vi "Modbus RTU Serial Request Translator.vi"(11 "请求字符串":string) -> (3 "转换后的字符串":string)   [LabVIEW 2014]
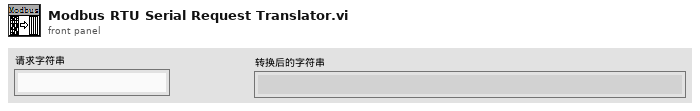
[diagram p1: front panel]
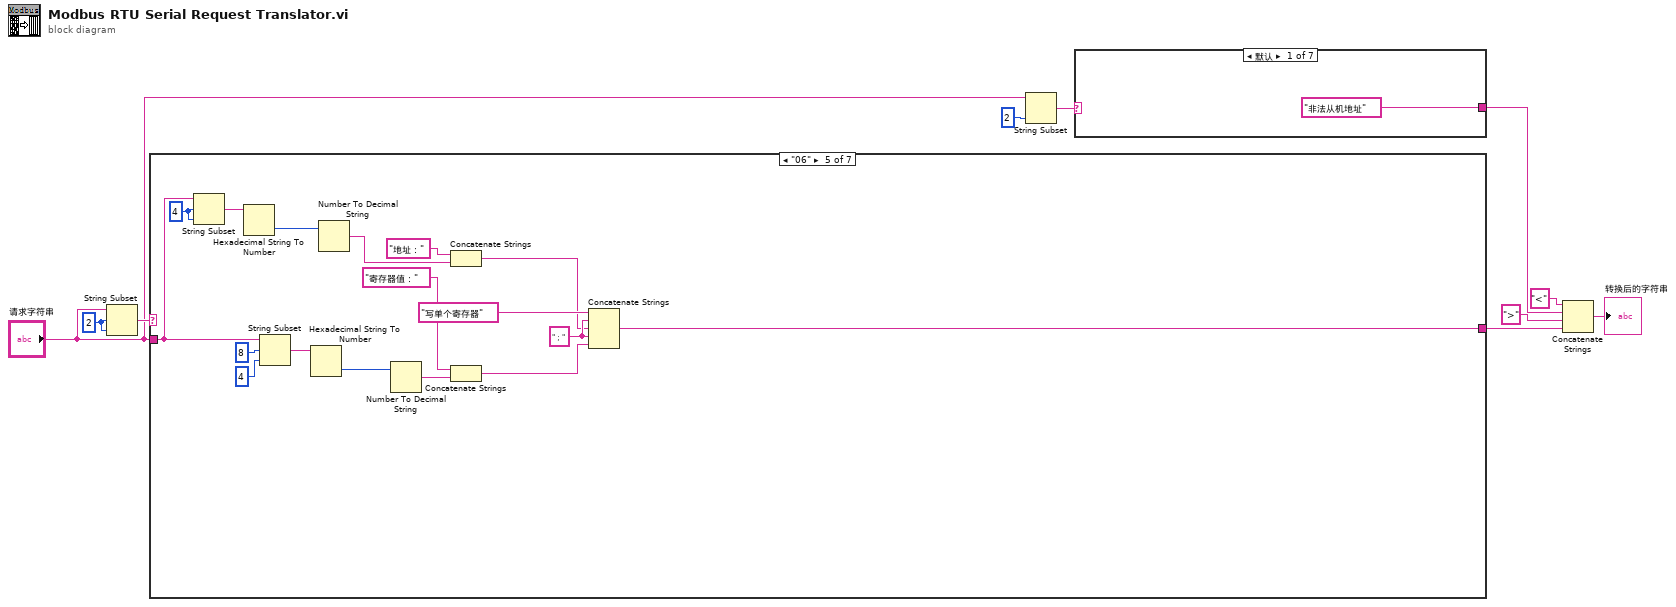
[diagram p0: block diagram]
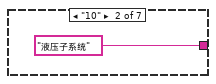
[diagram p2: hidden frame]
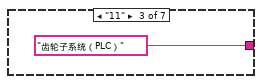
[diagram p3: hidden frame]
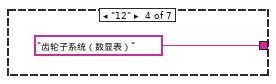
[diagram p4: hidden frame]
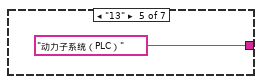
[diagram p5: hidden frame]
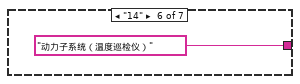
[diagram p6: hidden frame]
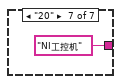
[diagram p7: hidden frame]
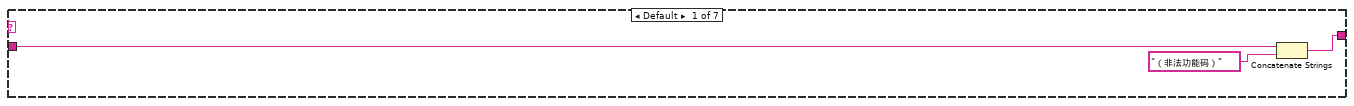
[diagram p8: hidden frame]
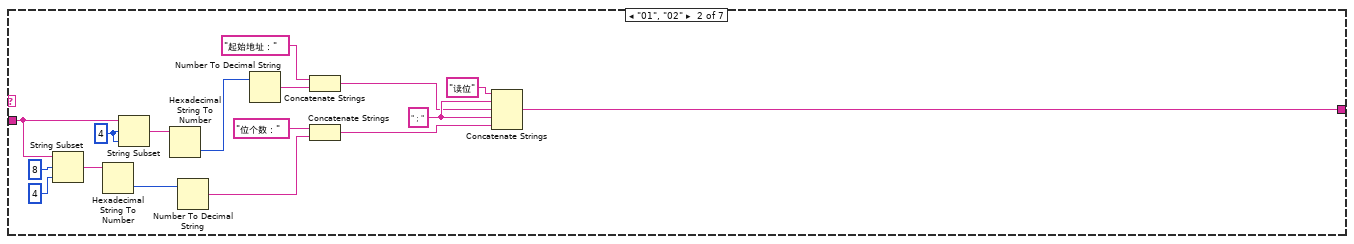
[diagram p9: hidden frame]
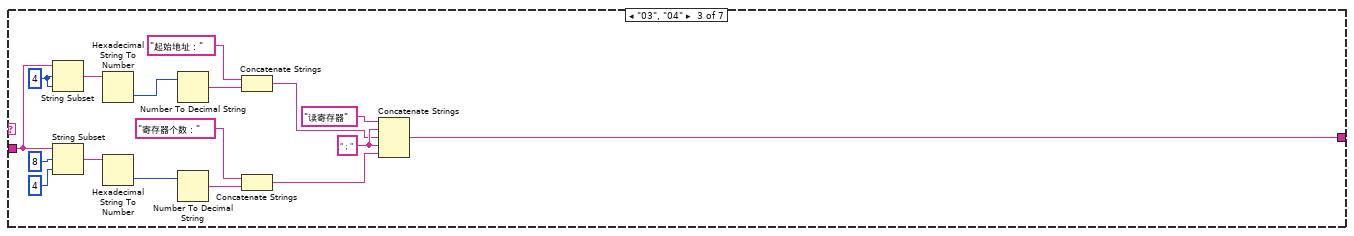
[diagram p10: hidden frame]
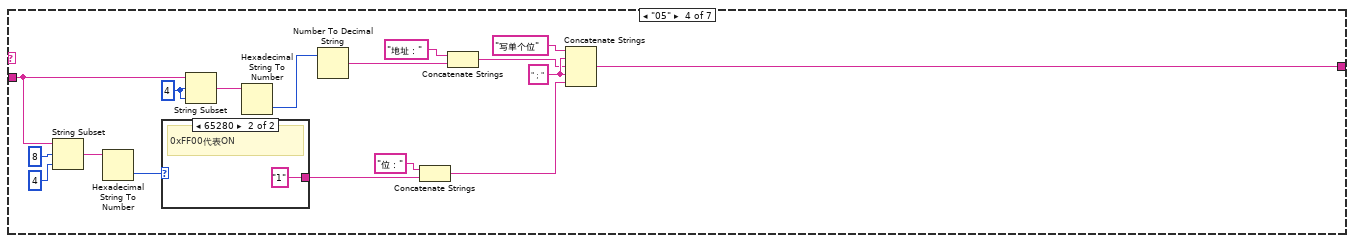
[diagram p11: hidden frame]
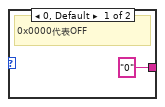
[diagram p12: hidden frame]
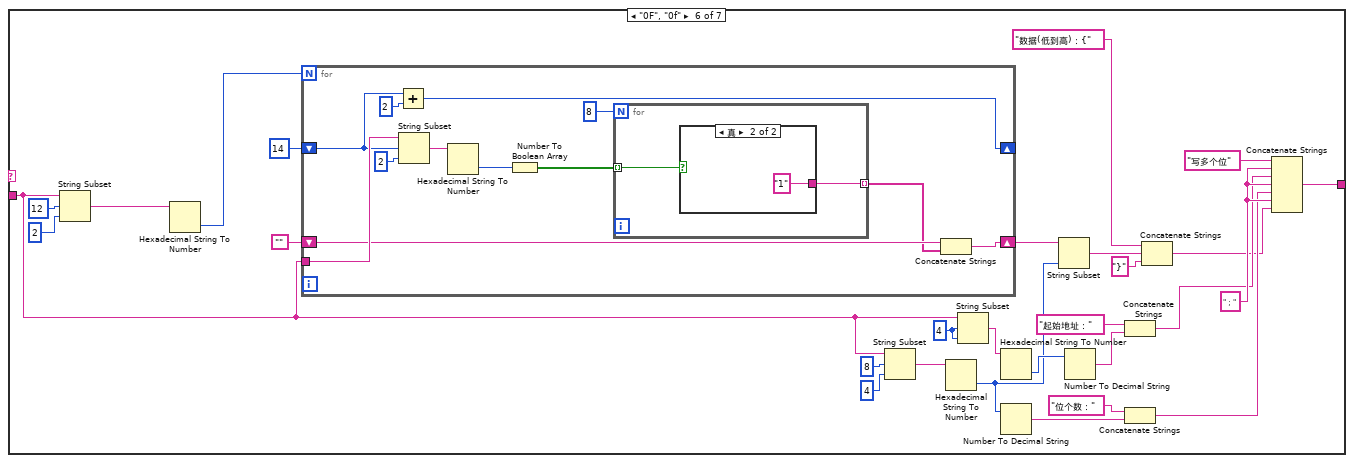
[diagram p13: hidden frame]
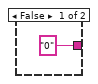
[diagram p14: hidden frame]
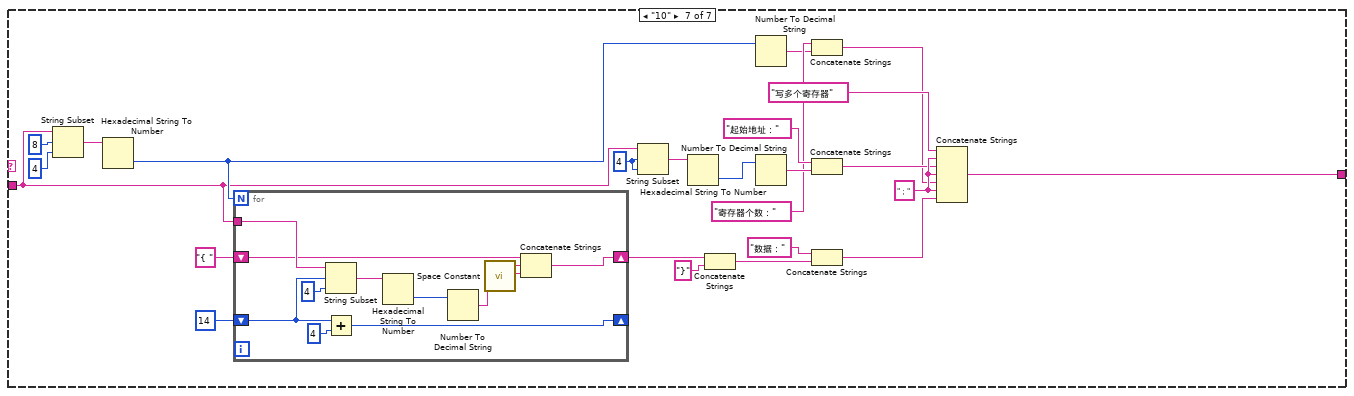
[diagram p15: hidden frame]
diagram:
  w10 = 2 ("偏移量(0)")
  n1 = String Subset(string="请求字符串", offset (0)=w10, length (rest)=w10) -> (substring=w9:string)
  n2 = case shown="\"06\"" w9 {
    tunnel: "请求字符串" -> [w13 w15 w46 w51 w72 w89 w143]
    tunnel: [w11 w14 w31 w50 w67 w94 w128] -> w5
    frame Default {
      n3 = Concatenate Strings(w13, "（非法功能码）") -> (w11:string)
    }
    frame "01", "02" {
      w18 = "；"
      w30 = 4 ("偏移量(0)")
      n4 = String Subset(string=w15, offset (0)=8 ("偏移量(0)"), length (rest)=4 ("长度（剩余）")) -> (substring=w21:string)
      n5 = Hexadecimal String To Number(string=w21) -> (number=w22:u32)  [unwired: 2 in, 1 out]
      n6 = String Subset(string=w15, offset (0)=w30, length (rest)=w30) -> (substring=w27:string)
      n7 = Hexadecimal String To Number(string=w27) -> (number=w26:u32)  [unwired: 2 in, 1 out]
      n8 = Number To Decimal String(number=w22) -> (decimal integer string=w20:string)  [unwired: 1 in]
      n9 = Number To Decimal String(number=w26) -> (decimal integer string=w24:string)  [unwired: 1 in]
      n10 = Concatenate Strings("起始地址：", w24) -> (w17:string)
      n11 = Concatenate Strings("位个数：", w20) -> (w16:string)
      n12 = Concatenate Strings("读位", w18, w17, w18, w16) -> (w14:string)
    }
    frame "03", "04" {
      w34 = "；"
      w47 = 4 ("偏移量(0)")
      n13 = String Subset(string=w46, offset (0)=w47, length (rest)=w47) -> (substring=w43:string)
      n14 = String Subset(string=w46, offset (0)=8 ("偏移量(0)"), length (rest)=4 ("长度（剩余）")) -> (substring=w37:string)
      n15 = Hexadecimal String To Number(string=w43) -> (number=w42:u32)  [unwired: 2 in, 1 out]
      n16 = Hexadecimal String To Number(string=w37) -> (number=w38:u32)  [unwired: 2 in, 1 out]
      n17 = Number To Decimal String(number=w42) -> (decimal integer string=w40:string)  [unwired: 1 in]
      n18 = Number To Decimal String(number=w38) -> (decimal integer string=w36:string)  [unwired: 1 in]
      n19 = Concatenate Strings("起始地址：", w40) -> (w33:string)
      n20 = Concatenate Strings("寄存器个数：", w36) -> (w32:string)
      n21 = Concatenate Strings("读寄存器", w34, w33, w34, w32) -> (w31:string)
    }
    frame "05" {
      w54 = "；"
      w64 = 4 ("偏移量(0)")
      n22 = String Subset(string=w51, offset (0)=8 ("偏移量(0)"), length (rest)=4 ("长度（剩余）")) -> (substring=w56:string)
      n23 = Hexadecimal String To Number(string=w56) -> (number=w49:u32)  [unwired: 2 in, 1 out]
      n24 = case shown="65280" w49 {
        tunnel: ["0" "1"] -> w48
        frame 0, Default {
          # "0x0000代表OFF"
        }
        frame 65280 {
          # "0xFF00代表ON"
        }
      }
      n25 = String Subset(string=w51, offset (0)=w64, length (rest)=w64) -> (substring=w61:string)
      n26 = Hexadecimal String To Number(string=w61) -> (number=w60:u32)  [unwired: 2 in, 1 out]
      n27 = Number To Decimal String(number=w60) -> (decimal integer string=w58:string)  [unwired: 1 in]
      n28 = Concatenate Strings("位：", w48) -> (w52:string)
      n29 = Concatenate Strings("地址：", w58) -> (w53:string)
      n30 = Concatenate Strings("写单个位", w54, w53, w54, w52) -> (w50:string)
    }
    frame "06" {
      w70 = "；"
      w83 = 4 ("偏移量(0)")
      n31 = String Subset(string=w72, offset (0)=w83, length (rest)=w83) -> (substring=w80:string)
      n32 = Hexadecimal String To Number(string=w80) -> (number=w79:u32)  [unwired: 2 in, 1 out]
      n33 = String Subset(string=w72, offset (0)=8 ("偏移量(0)"), length (rest)=4 ("长度（剩余）")) -> (substring=w74:string)
      n34 = Hexadecimal String To Number(string=w74) -> (number=w75:u32)  [unwired: 2 in, 1 out]
      n35 = Number To Decimal String(number=w79) -> (decimal integer string=w77:string)  [unwired: 1 in]
      n36 = Number To Decimal String(number=w75) -> (decimal integer string=w73:string)  [unwired: 1 in]
      n37 = Concatenate Strings("地址：", w77) -> (w69:string)
      n38 = Concatenate Strings("寄存器值：", w73) -> (w68:string)
      n39 = Concatenate Strings("写单个寄存器", w70, w69, w70, w68) -> (w67:string)
    }
    frame "0F", "0f" {
      w99 = "；"
      w111 = 4 ("偏移量(0)")
      n40 = String Subset(string=w89, offset (0)=12 ("偏移量(0)"), length (rest)=2 ("长度（剩余）")) -> (substring=w91:string)
      n41 = Hexadecimal String To Number(string=w91) -> (number=w90:u32)  [unwired: 2 in, 1 out]
      n42 = for {
        N: w90 -> [_]
        shift-right: [w123] -> _
        shift-left: 14 ("偏移量(0)") -> [w120]
        tunnel: w89 -> [w121]
        shift-right: [w116] -> w86
        shift-left: "" -> [w117]
        n43 = Add(x=w120, y=2) -> (x+y=w123:i32)
        n44 = String Subset(string=w121, offset (0)=w120, length (rest)=2 ("长度（剩余）")) -> (substring=w118:string)
        n45 = Hexadecimal String To Number(string=w118) -> (number=w115:u32)  [unwired: 2 in, 1 out]
        n46 = Number To Boolean Array(number=w115) -> (Boolean array=w113:bool[])
        n47 = for {
          N: 8 -> [_]
          tunnel: w113 -> [w125] mode=indexing
          tunnel: [w124] -> w112 mode=indexing
          n48 = case shown="真" w125 {
            tunnel: ["0" "1"] -> w124
            frame False {
            }
            frame True {
            }
          }
        }
        n49 = Concatenate Strings(w117, w112) -> (w116:string)
      }
      n50 = String Subset(string=w89, offset (0)=8 ("偏移量(0)"), length (rest)=4 ("长度（剩余）")) -> (substring=w106:string)
      n51 = Hexadecimal String To Number(string=w106) -> (number=w84:u32)  [unwired: 2 in, 1 out]
      n52 = String Subset(string=w89, offset (0)=w111, length (rest)=w111) -> (substring=w108:string)
      n53 = Hexadecimal String To Number(string=w108) -> (number=w107:u32)  [unwired: 2 in, 1 out]
      n54 = Number To Decimal String(number=w84) -> (decimal integer string=w101:string)  [unwired: 1 in]
      n55 = String Subset(string=w86, length (rest)=w84) -> (substring=w85:string)  [unwired: 1 in]
      n56 = Number To Decimal String(number=w107) -> (decimal integer string=w103:string)  [unwired: 1 in]
      n57 = Concatenate Strings("起始地址：", w103) -> (w97:string)
      n58 = Concatenate Strings("位个数：", w101) -> (w96:string)
      n59 = Concatenate Strings("数据(低到高)：{", w85, "}" ("字符串")) -> (w95:string)
      n60 = Concatenate Strings("写多个位", w99, w97, w99, w96, w99, w95) -> (w94:string)
    }
    frame "10" {
      w133 = "；"
      w151 = 4 ("偏移量(0)")
      n61 = String Subset(string=w143, offset (0)=8 ("偏移量(0)"), length (rest)=4 ("长度（剩余）")) -> (substring=w146:string)
      n62 = Hexadecimal String To Number(string=w146) -> (number=w144:u32)  [unwired: 2 in, 1 out]
      n63 = for {
        N: w144 -> [_]
        shift-right: [w162] -> _
        shift-left: 14 ("偏移量(0)") -> [w159]
        tunnel: w143 -> [w160]
        shift-right: [w152] -> w141
        shift-left: "{ " -> [w155]
        n64 = String Subset(string=w160, offset (0)=w159, length (rest)=4 ("长度（剩余）")) -> (substring=w157:string)
        n65 = Add(x=w159, y=4) -> (x+y=w162:i32)
        n66 = Hexadecimal String To Number(string=w157) -> (number=w156:u32)  [unwired: 2 in, 1 out]
        n67 = Number To Decimal String(number=w156) -> (decimal integer string=w154:string)  [unwired: 1 in]
        n68 = call <vilib>:"Space Constant.vi"() -> ("String"=w153:string)
        n69 = Concatenate Strings(w155, w154, w153) -> (w152:string)
      }
      n70 = String Subset(string=w143, offset (0)=w151, length (rest)=w151) -> (substring=w148:string)
      n71 = Hexadecimal String To Number(string=w148) -> (number=w147:u32)  [unwired: 2 in, 1 out]
      n72 = Concatenate Strings(w141, "}" ("字符串")) -> (w134:string)
      n73 = Number To Decimal String(number=w144) -> (decimal integer string=w136:string)  [unwired: 1 in]
      n74 = Number To Decimal String(number=w147) -> (decimal integer string=w138:string)  [unwired: 1 in]
      n75 = Concatenate Strings("寄存器个数：", w136) -> (w130:string)
      n76 = Concatenate Strings("起始地址：", w138) -> (w131:string)
      n77 = Concatenate Strings("数据：", w134) -> (w129:string)
      n78 = Concatenate Strings("写多个寄存器", w133, w131, w133, w130, w133, w129) -> (w128:string)
    }
  }
  n79 = String Subset(string="请求字符串", length (rest)=2 ("长度（剩余）")) -> (substring=w8:string)  [unwired: 1 in]
  n80 = case shown="默认" w8 {
    tunnel: ["非法从机地址" "液压子系统" "齿轮子系统（PLC）" "齿轮子系统（数显表）" "动力子系统（PLC）" "动力子系统（温度巡检仪）" "NI工控机"] -> w2
    frame Default {
    }
    frame "10" {
    }
    frame "11" {
    }
    frame "12" {
    }
    frame "13" {
    }
    frame "14" {
    }
    frame "20" {
    }
  }
  n81 = Concatenate Strings("<" ("字符串"), w2, ">" ("字符串"), w5) -> (→"转换后的字符串":string)
